vi "Projekt_zamek_szyfrowy.vi"() -> ()   [LabVIEW 2023]
panel:
  in  "Lock_data":string[][](array[string])=[["Admin", "1234"], ["Mama", "2345"], ["Tata", "3456"], ["Brat", "4567"]]
  out "String 2":string
  in  "Show password":bool
  out "Password":string
  out "Slide":u8(slide) scale=0.0..100.0
  in  "Numpad":T1
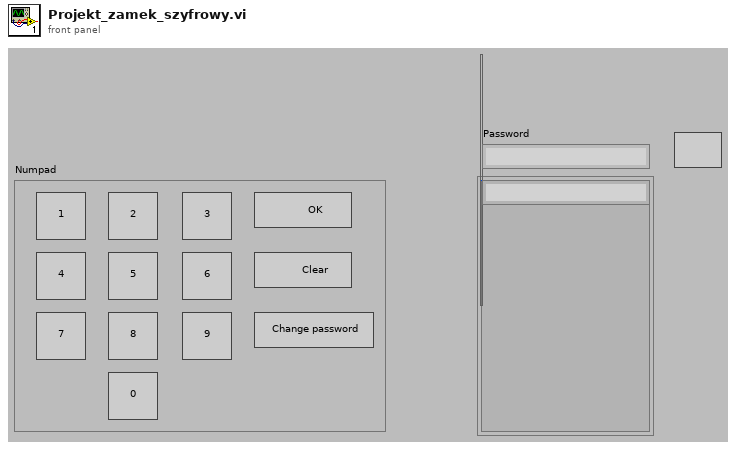
[diagram p1: front panel]
types:
  T1 = cluster{"Blank Button":bool, "Blank Button 2":bool, "Blank Button 3":bool, "Blank Button 4":bool, "Blank Button 5":bool, "Blank Button 6":bool, "Blank Button 7":bool, "Blank Button 8":bool, "Blank Button 9":bool, "Blank Button 10":bool, "OK Button":bool, "Clear button":bool, "Change password button":bool}
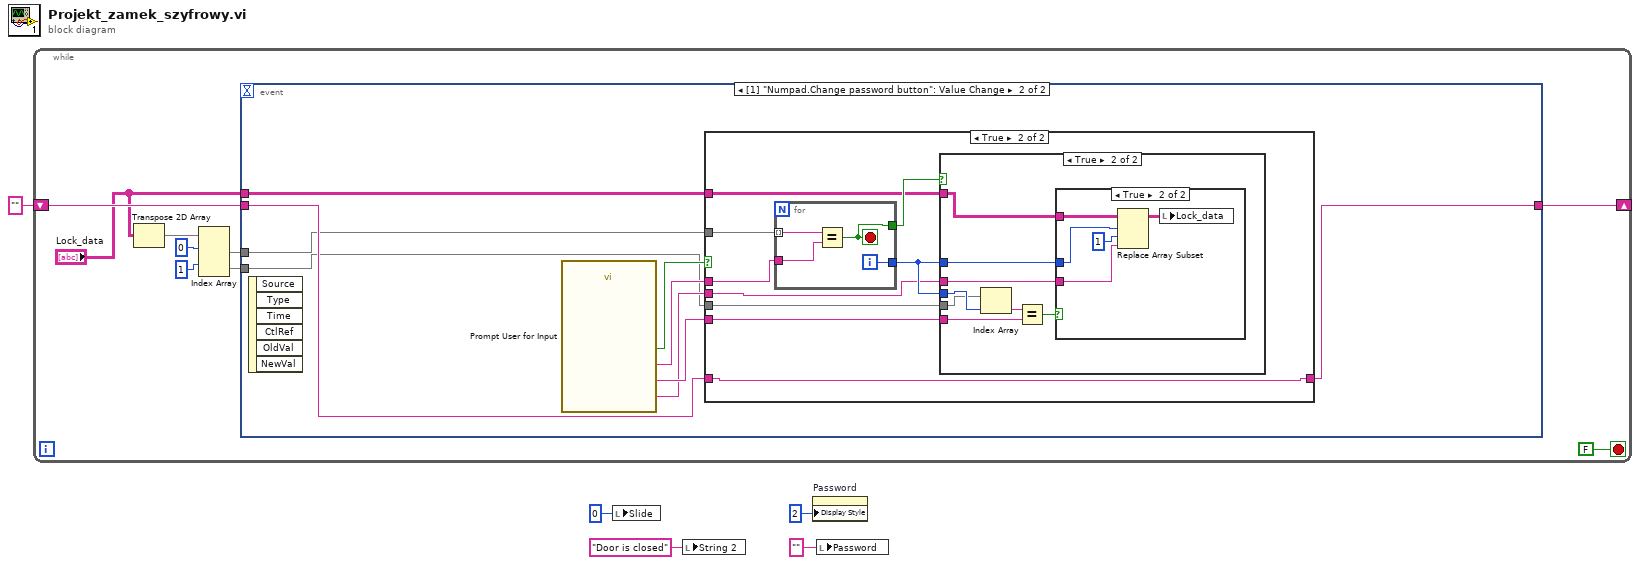
[diagram p0: block diagram]
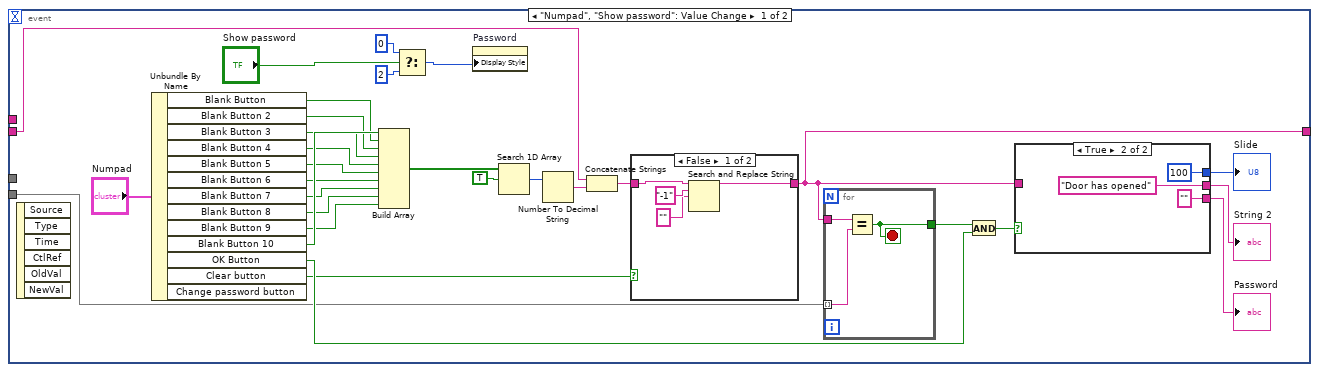
[diagram p2: hidden frame]
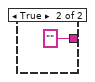
[diagram p3: hidden frame]
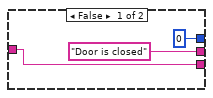
[diagram p4: hidden frame]
diagram:
  n1 = while {
    shift-right: [w14] -> _
    shift-left: "" -> [w13]
    stop <- FALSE stop-if-true
    n2 = Transpose 2D Array(2D array="Lock_data") -> (transposed array=w12:string[][])
    n3 = Index Array(array=w12, index (row) #1=0 ("index (row)"), index (row) #2=1 ("index (row)")) -> (element #1=w9:string[], element #2=w8:string[])  [unwired: 2 in]
    n4 = event shown="[1] \"Numpad.Change password button\": Value Change" {
      selector: _ -> [_ _]
      dyn-events: _ -> [_ _]
      timeout: _ -> [_ _]
      tunnel: [w20 w66] -> w14
      tunnel: w13 -> [w29 w67]
      tunnel: w9 -> [_ w61]
      tunnel: w8 -> [w15 w60]
      tunnel: "Lock_data" -> [_ w59]
      event "Numpad", "Show password": Value Change {
        n5 = event-data() -> ()  [unwired: 1 in, 6 out]
        n6 = Unbundle By Name("Numpad") -> ("Blank Button"=w42:bool, "Blank Button 2"=w34:bool, "Blank Button 3"=w41:bool, "Blank Button 4"=w40:bool, "Blank Button 5"=w39:bool, "Blank Button 6"=w38:bool, "Blank Button 7"=w37:bool, "Blank Button 8"=w36:bool, "Blank Button 9"=w35:bool, "Blank Button 10"=w43:bool, "OK Button"=w25:bool, "Clear button"=w22:bool)  [unwired: 1 out]
        n7 = Build Array(w43, w42, w34, w41, w40, w39, w38, w37, w36, w35) -> (w33:bool[])
        n8 = Select(t=u32 0 ("Display Style"), s="Show password", f=2) -> (s? t:f=w16:u32)
        n9 = property on="Password" class="Str"("Display Style"=w16) -> ()  [unwired: 2 in, 2 out]
        n10 = Search 1D Array(1D array=w33, element=TRUE) -> (index of element=w31:i32)  [unwired: 1 in]
        n11 = Number To Decimal String(number=w31) -> (decimal integer string=w30:string)  [unwired: 1 in]
        n12 = Concatenate Strings(w29, w30) -> (w23:string)
        n13 = case shown="False" w22 {
          tunnel: w23 -> [w49 _]
          tunnel: [w48 ""] -> w20
          frame False {
            n14 = Search and Replace String(input string=w49, search string="-1", replace string="" ("replace string (\"\")")) -> (result string=w48:string)  [unwired: 5 in, 3 out]
          }
          frame True {
          }
        }
        n15 = for {
          tunnel: [w45] -> w26
          tunnel: w20 -> [w47]
          tunnel: w15 -> [w46] mode=indexing
          stop <- w45 stop-if-true
          n16 = Equal?(x=w47, y=w46) -> (x = y?=w45:bool)
        }
        n17 = And(x=w26, y=w25) -> (x .and. y?=w24:bool)
        n18 = case shown="True" w24 {
          tunnel: [u8 0 ("Slide") u8 100 ("Slide")] -> w28
          tunnel: ["Door is closed" ("String 2") "Door has opened" ("String 2")] -> w27
          tunnel: w20 -> [w53 _]
          tunnel: [w53 ""] -> w21
          frame False {
          }
          frame True {
          }
        }
        "Slide" <- w28
        "String 2" <- w27
        "Password" <- w21
      }
      event "Numpad.Change password button": Value Change {
        n19 = event-data() -> ()  [unwired: 1 in, 6 out]
        n20 = call "Prompt User for Input"() -> ("New password"=w62:string, "password"=w63:string, "User"=w64:string, "OK"=w65:bool)  [unwired: 15 in, 1 out]
        n21 = case shown="True" w65 {
          tunnel: w67 -> [w68 w77]
          tunnel: [w68 w77] -> w66
          tunnel: w64 -> [_ w75]
          tunnel: w63 -> [_ w73]
          tunnel: w62 -> [_ w70]
          tunnel: w61 -> [_ w76]
          tunnel: w60 -> [_ w74]
          tunnel: w59 -> [_ w69]
          frame False {
          }
          frame True {
            n22 = for {
              tunnel: [w92] -> w72
              tunnel: w76 -> [w94] mode=indexing
              tunnel: w75 -> [w93]
              tunnel: [w91] -> w71
              i -> [w91]
              stop <- w92 stop-if-true
              n23 = Equal?(x=w94, y=w93) -> (x = y?=w92:bool)
            }
            n24 = case shown="True" w72 {
              tunnel: w71 -> [_ w85]
              tunnel: w74 -> [_ w84]
              tunnel: w73 -> [_ w82]
              tunnel: w71 -> [_ w80]
              tunnel: w70 -> [_ w79]
              tunnel: w69 -> [_ w78]
              frame False {
              }
              frame True {
                n25 = Index Array(array=w84, index=w85) -> (element=w83:string)
                n26 = Equal?(x=w83, y=w82) -> (x = y?=w81:bool)
                n27 = case shown="True" w81 {
                  tunnel: w80 -> [_ w88]
                  tunnel: w79 -> [_ w90]
                  tunnel: w78 -> [_ w89]
                  frame False {
                  }
                  frame True {
                    n28 = Replace Array Subset(array=w89, new element=w90, index (row)=w88, index (col)=1 ("disabled index (col)")) -> (w86:string[][])
                    n29 = local write "Lock_data"(w86) -> ()
                  }
                }
              }
            }
          }
        }
      }
    }
  }
  n30 = local write "Slide"(u8 0 ("Slide")) -> ()
  n31 = local write "String 2"("Door is closed" ("String 2")) -> ()
  n32 = property on="Password" class="Str"("Display Style"=2) -> ()  [unwired: 2 in, 2 out]
  n33 = local write "Password"("" ("Password")) -> ()
